vi "Set Initialization Data - UGM BEEP.vi"(8 "error in":errorcluster, 11 "Controller in":refnum<class "Controller.lvclass">) -> (0 "error out":errorcluster, 3 "Controller out":refnum<class "Controller.lvclass">)   [LabVIEW 2024, in "Controller.lvclass"]
doc: "In this VI you can set the initialization data of a statically-linked subWorker."
uses:
  Controller.lvclass
  Controller.lvclass/Controller.ctl
  UGM BEEP/Initialization Data.ctl
  UGM BEEP/UGM BEEP.lvclass
  C:/Program Files (x86)/National Instruments/LabVIEW 2024/vi.lib/addons/_Workers/Library/Classes/Worker/Worker.lvclass
  C:/Program Files (x86)/National Instruments/LabVIEW 2024/vi.lib/addons/_Workers/Library/Classes/Workers Object/Workers Object.lvclass
  C:/_Repo/ugm24-dp2/src/Workers/UGM BEEP/UGM BEEP.lvclass
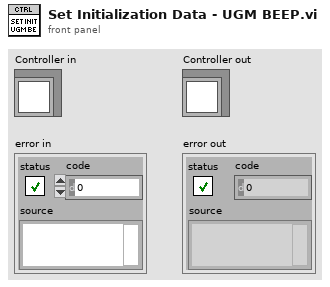
[diagram p1: front panel]
types:
  T1 = typedef "UGM BEEP.lvclass/Initialization Data.ctl" = cluster{"String":string}
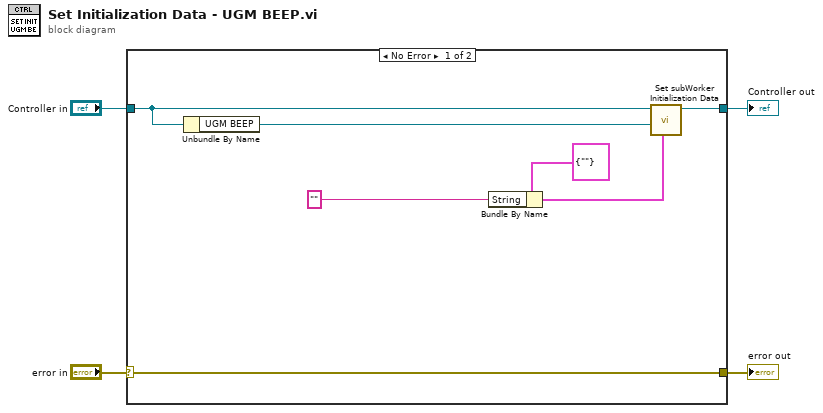
[diagram p0: block diagram]
diagram:
  n1 = case shown="No Error" "error in" {
    selector: "error in" -> [w11 w13]
    tunnel: [w11 w13] -> w3
    tunnel: [w9 w12] -> w2
    tunnel: "Controller in" -> [w8 w12]
    frame No Error {
      n2 = Unbundle By Name(w8) -> ("UGM BEEP"=w10:refnum<class "UGM BEEP.lvclass">)
      n3 = Bundle By Name(cluster=T1 {"String"=""} ("Initialization Data"), "String"="" ("Placeholder")) -> (w6:T1)
      n4 = call-dynamic "Set subWorker Initialization Data.vi"("Initialization Data"=w6, "subWorker"=w10, "Worker"=w8) -> ("Worker out"=w9:refnum<class "Controller.lvclass">)  [unwired: 8 in]
    }
    frame Error {
    }
  }
  "error out" <- w3
  "Controller out" <- w2
